vi "CHECK_STOCK.vi"(10 "CURRENT_YEAR_DATA":string, 11 "connection reference":T1) -> ()   [LabVIEW 2015]
uses:
  Controls/CHECK_STOCK.ctl
  <vilib>/addons/database/Connection.llb/Conn ObjectReference.ctl
  <vilib>/Utility/miscctls.llb/LVRowAndColumnUnsignedTypeDef.ctl
  Controls/ITEM_CODE_CLUSTER.ctl
  Controls/STORE_INITAIL_INFORMATION.ctl
  <vilib>/Utility/error.llb/DialogType.ctl
  <vilib>/addons/database/Connection.llb/Conn Execute.vi
  <vilib>/addons/database/Recordset.llb/Rec Destroy - Connection.vi
  <vilib>/addons/database/_DB Variant To Data/Database Variant To Data.xnode
  <vilib>/addons/database/NI_Database_API.lvlib
  <vilib>/addons/database/Connection.llb/DB Tools Open Connec (String).vi
panel:
  out "COUNTER":i32
  out "Find Array":i32[](array[numeric])
  in  "Next Button":bool
  in  "SEARCH":string
  in  "END_MONTH Button":bool
  out "Array":T2[](array[typedef])
  in  "BOTTON_IMPORT":bool
  in  "BUTTON_EXIT":bool
  in  "Tab Control":enum32{"FROM CHECK STOCK", "TRANSFER"}(tab)
  in  "PRODUCT":string(combo)
  in  "INITAIL DATE FROM":string(combo) caption="DATE FROM"
  in  "TO":string(combo)
  in  "TRANFER_DATE_FROM":timestamp caption="DATE (FROM)" format="%<%Y>T"
  in  "(TO)":timestamp format="%<%Y>T"
  out "Table":string[][](table)
  # "CHECK STOCK"
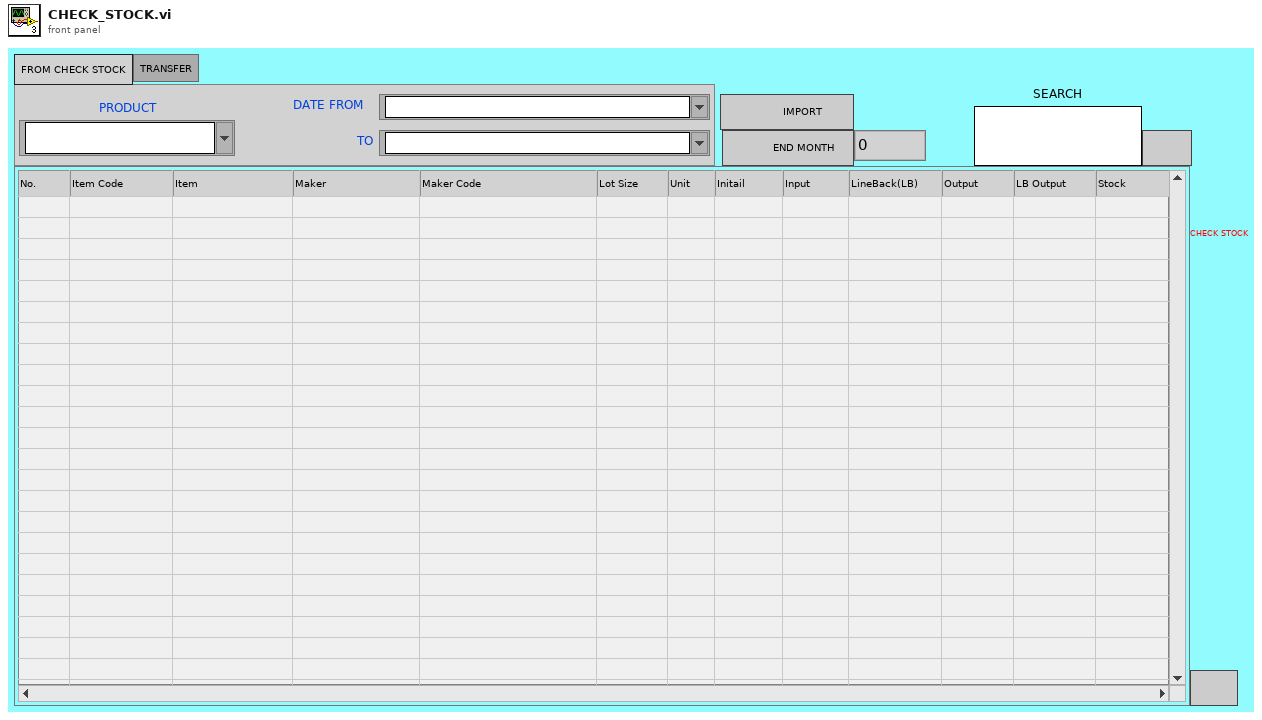
[diagram p1: front panel]
types:
  T1 = typedef "NI_Database_API.lvlib/Conn ObjectReference.ctl" = refnum<k1>
  T2 = typedef "CHECK_STOCK.ctl" = cluster{"ITEM_CODE":string, "PART_NAME":string, "MAKER":string, "PART_NO":string, "LOT_SIZE":dbl, "UNIT":string, "INITAIL":dbl, "INPUT":dbl, "OUTPUT":dbl, "LINEBACK":dbl, "LINEBACK_OUTPUT":dbl, "STOCK":dbl}
  T3 = typedef "LVRowAndColumnUnsignedTypeDef.ctl" = cluster{"Row":u32, "Column":u32}
  T4 = typedef "ITEM_CODE_CLUSTER.ctl" = cluster{"ITEM_CODE":string, "INVOICE_NO":string, "INVOICE_DATE":timestamp, "LOT_MAKER":string, "QUANTITY":dbl, "INVOICE_ECODE":string, "INPUT_NO":string, "INPUT_DATE":timestamp, "INPUT_ECODE":string, "LINEBACK_NO":string, "LINEBACK_DATE":timestamp, "LINEBACK_ECODE":string, "OUTPUT_NO":string, "OUTPUT_DATE":timestamp, "OUTPUT_ECODE":string, "DESTINATION":string}
  T5 = typedef "STORE_INITAIL_INFORMATION.ctl" = cluster{"DATE":timestamp, "PRODUCT":string, "NO":string, "ECODE":string}
  T6 = typedef "NI_Database_API.lvlib/Rec ObjectReference.ctl" = refnum<k1>
  T7 = typedef "DialogType.ctl" = u16
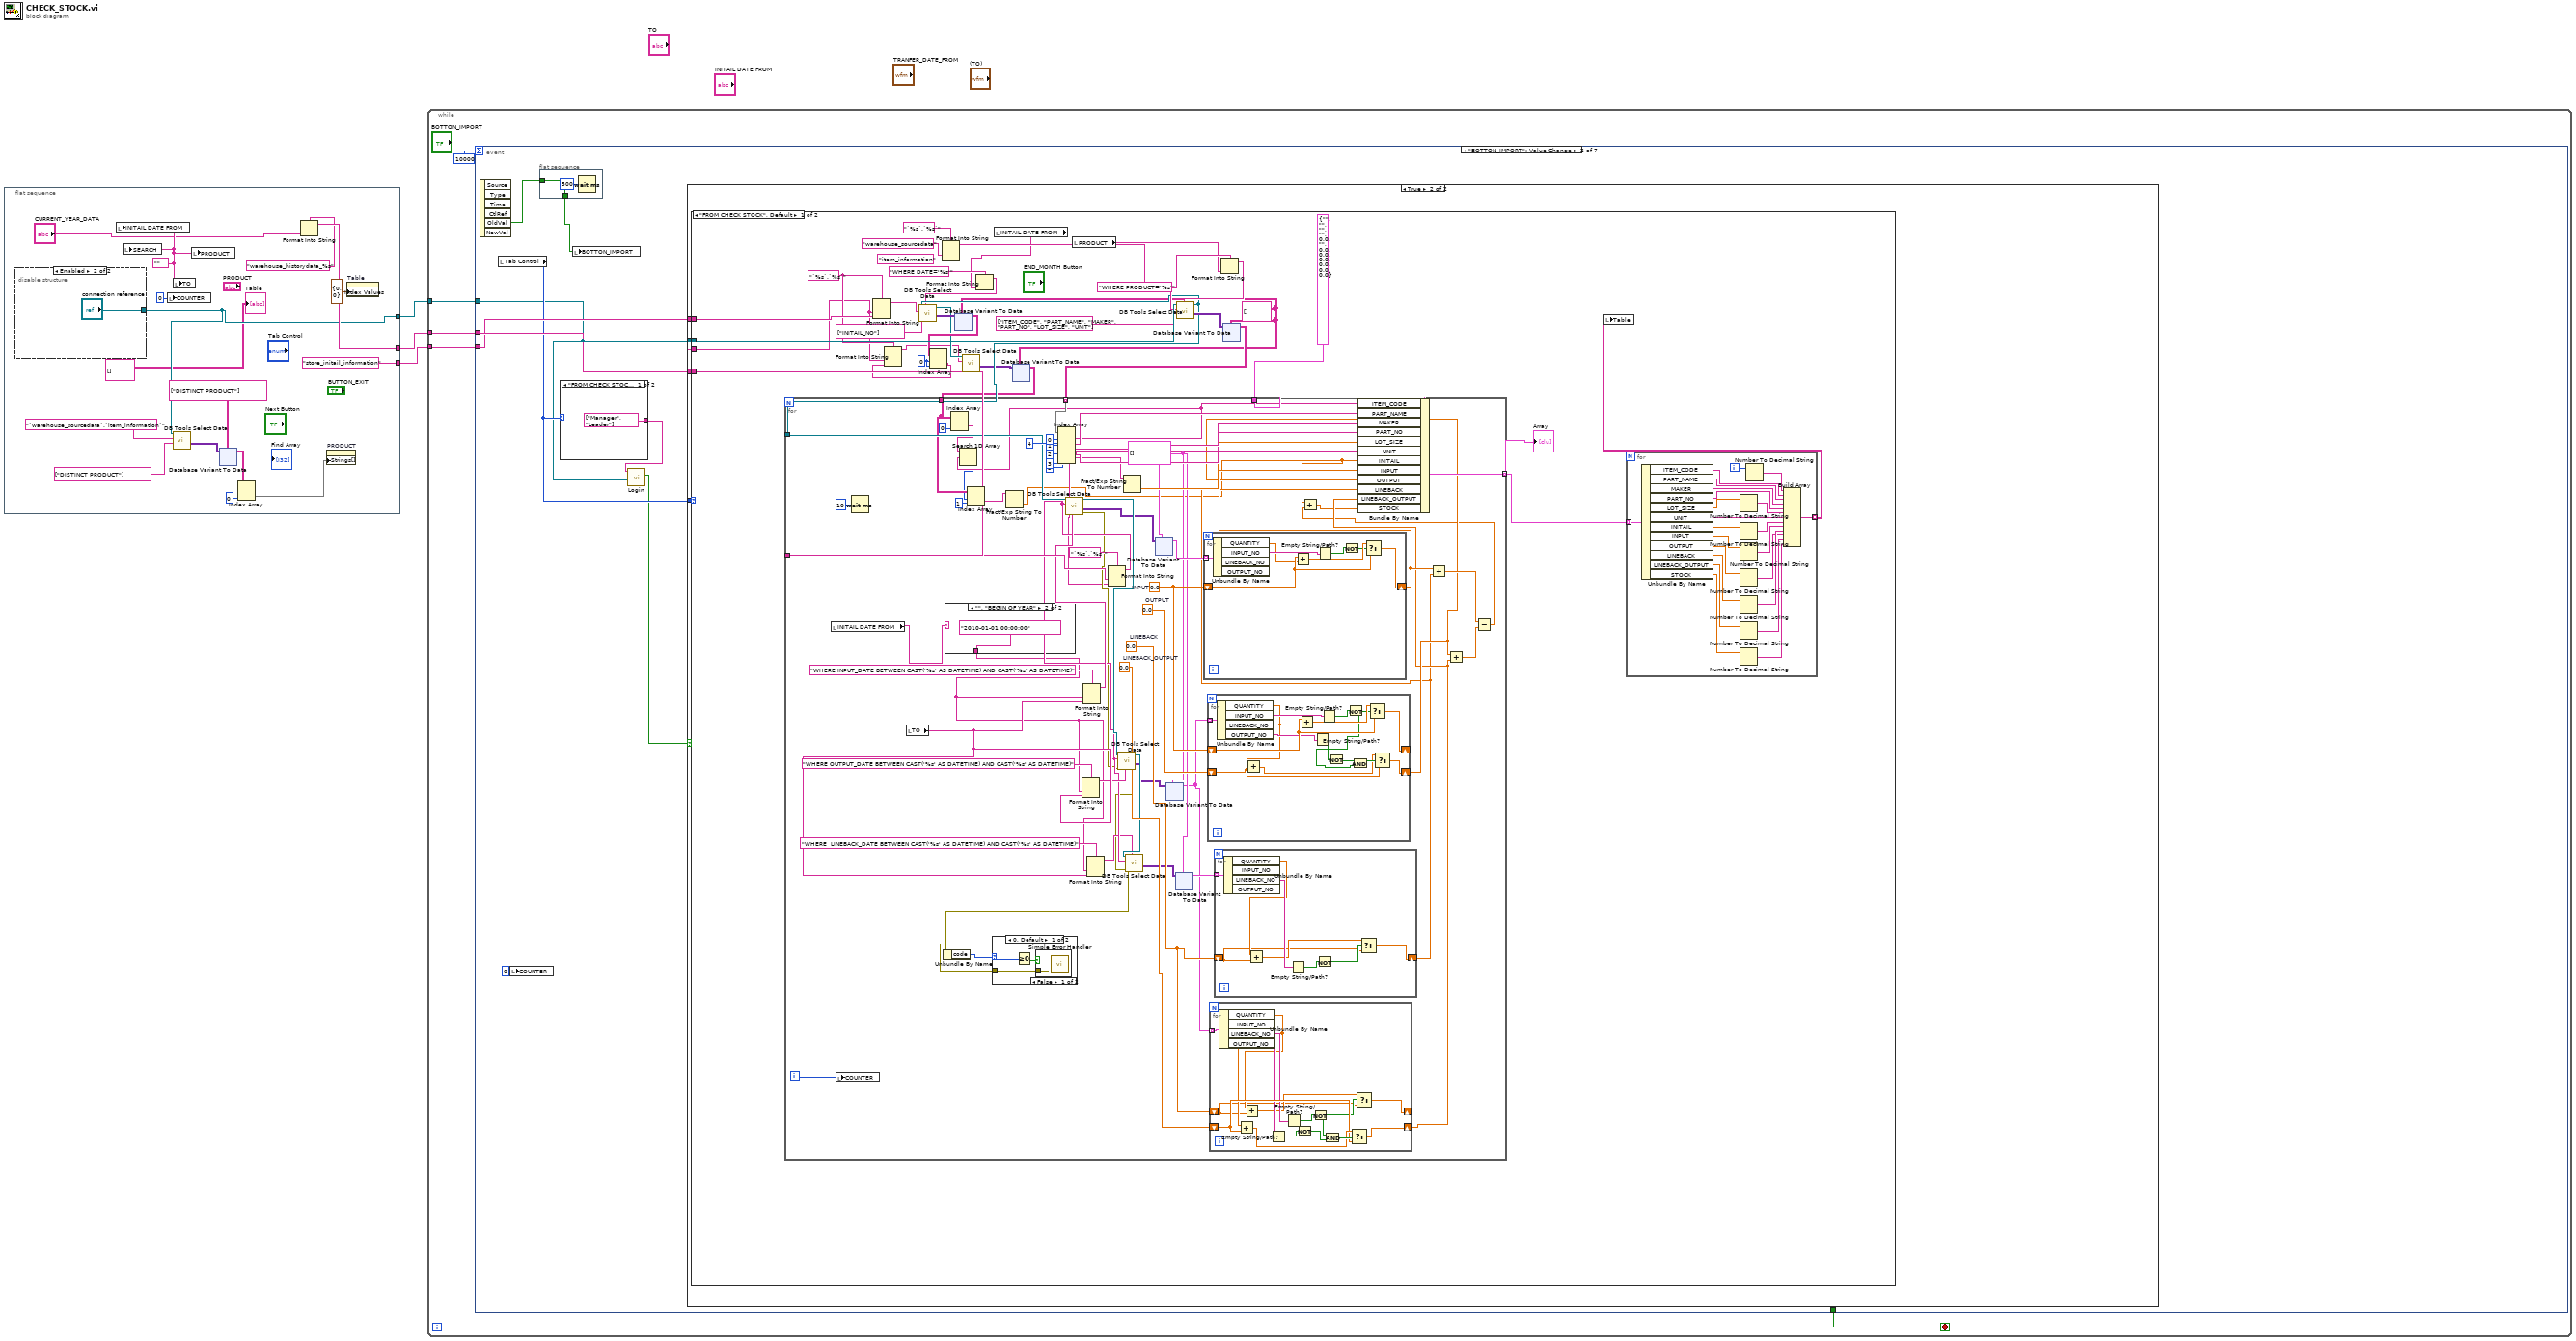
[diagram p0: block diagram]
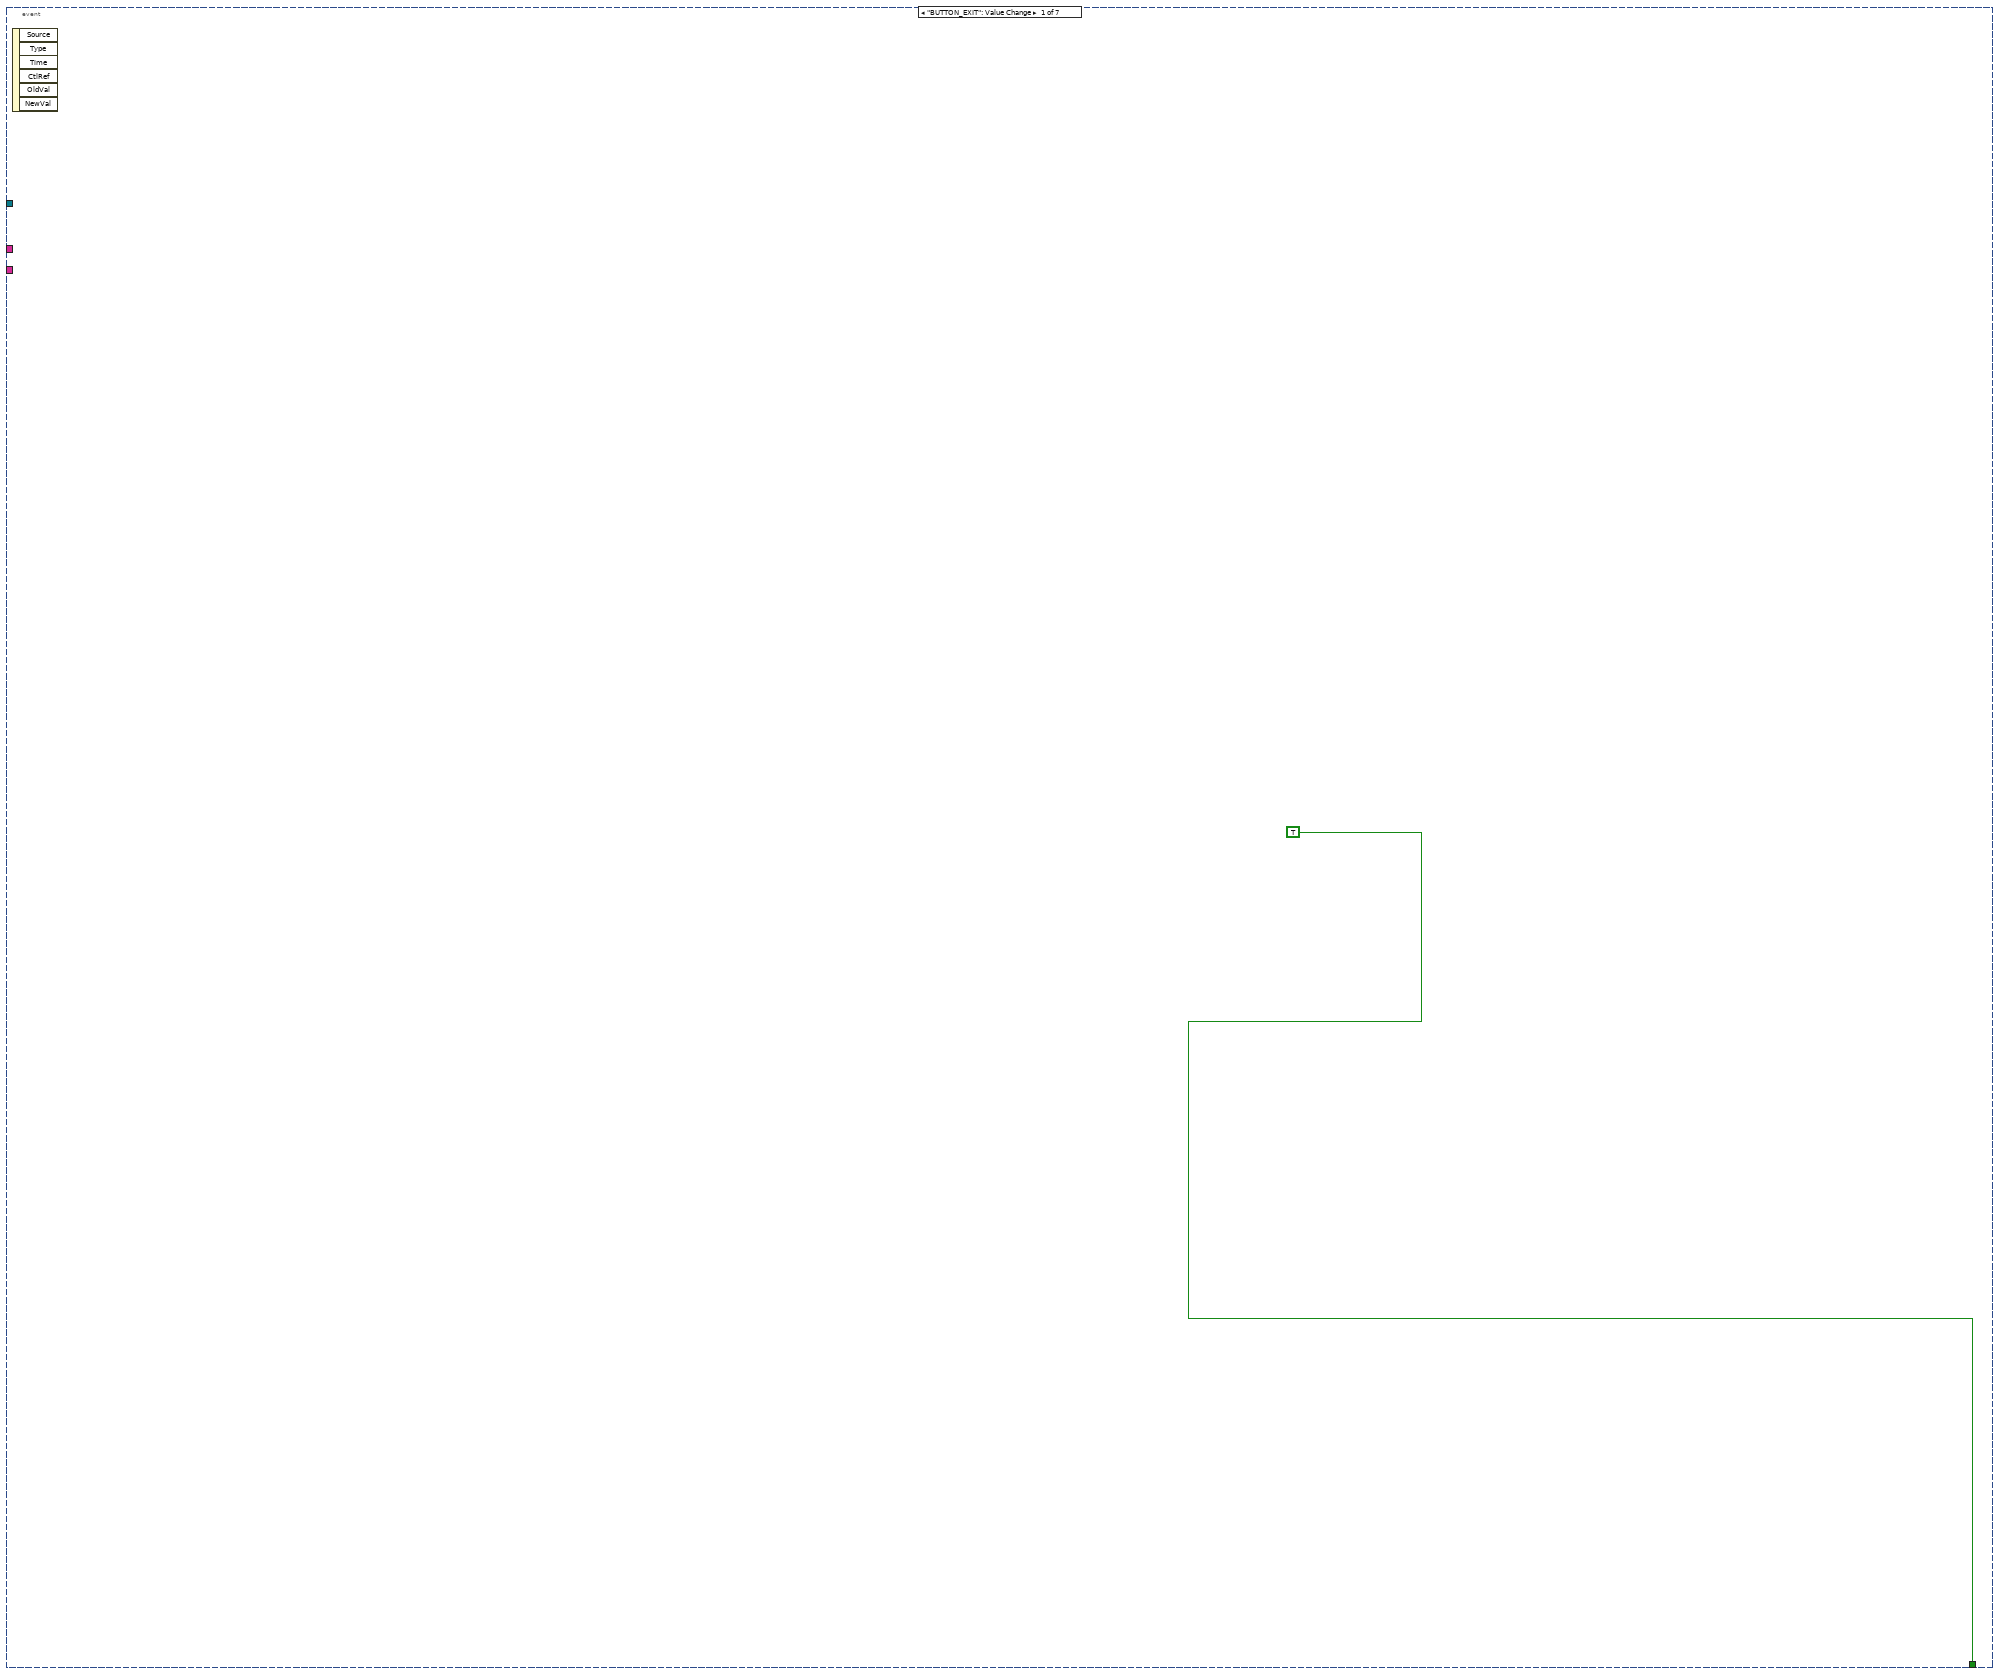
[diagram p2: hidden frame]
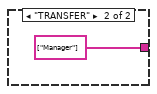
[diagram p3: hidden frame]
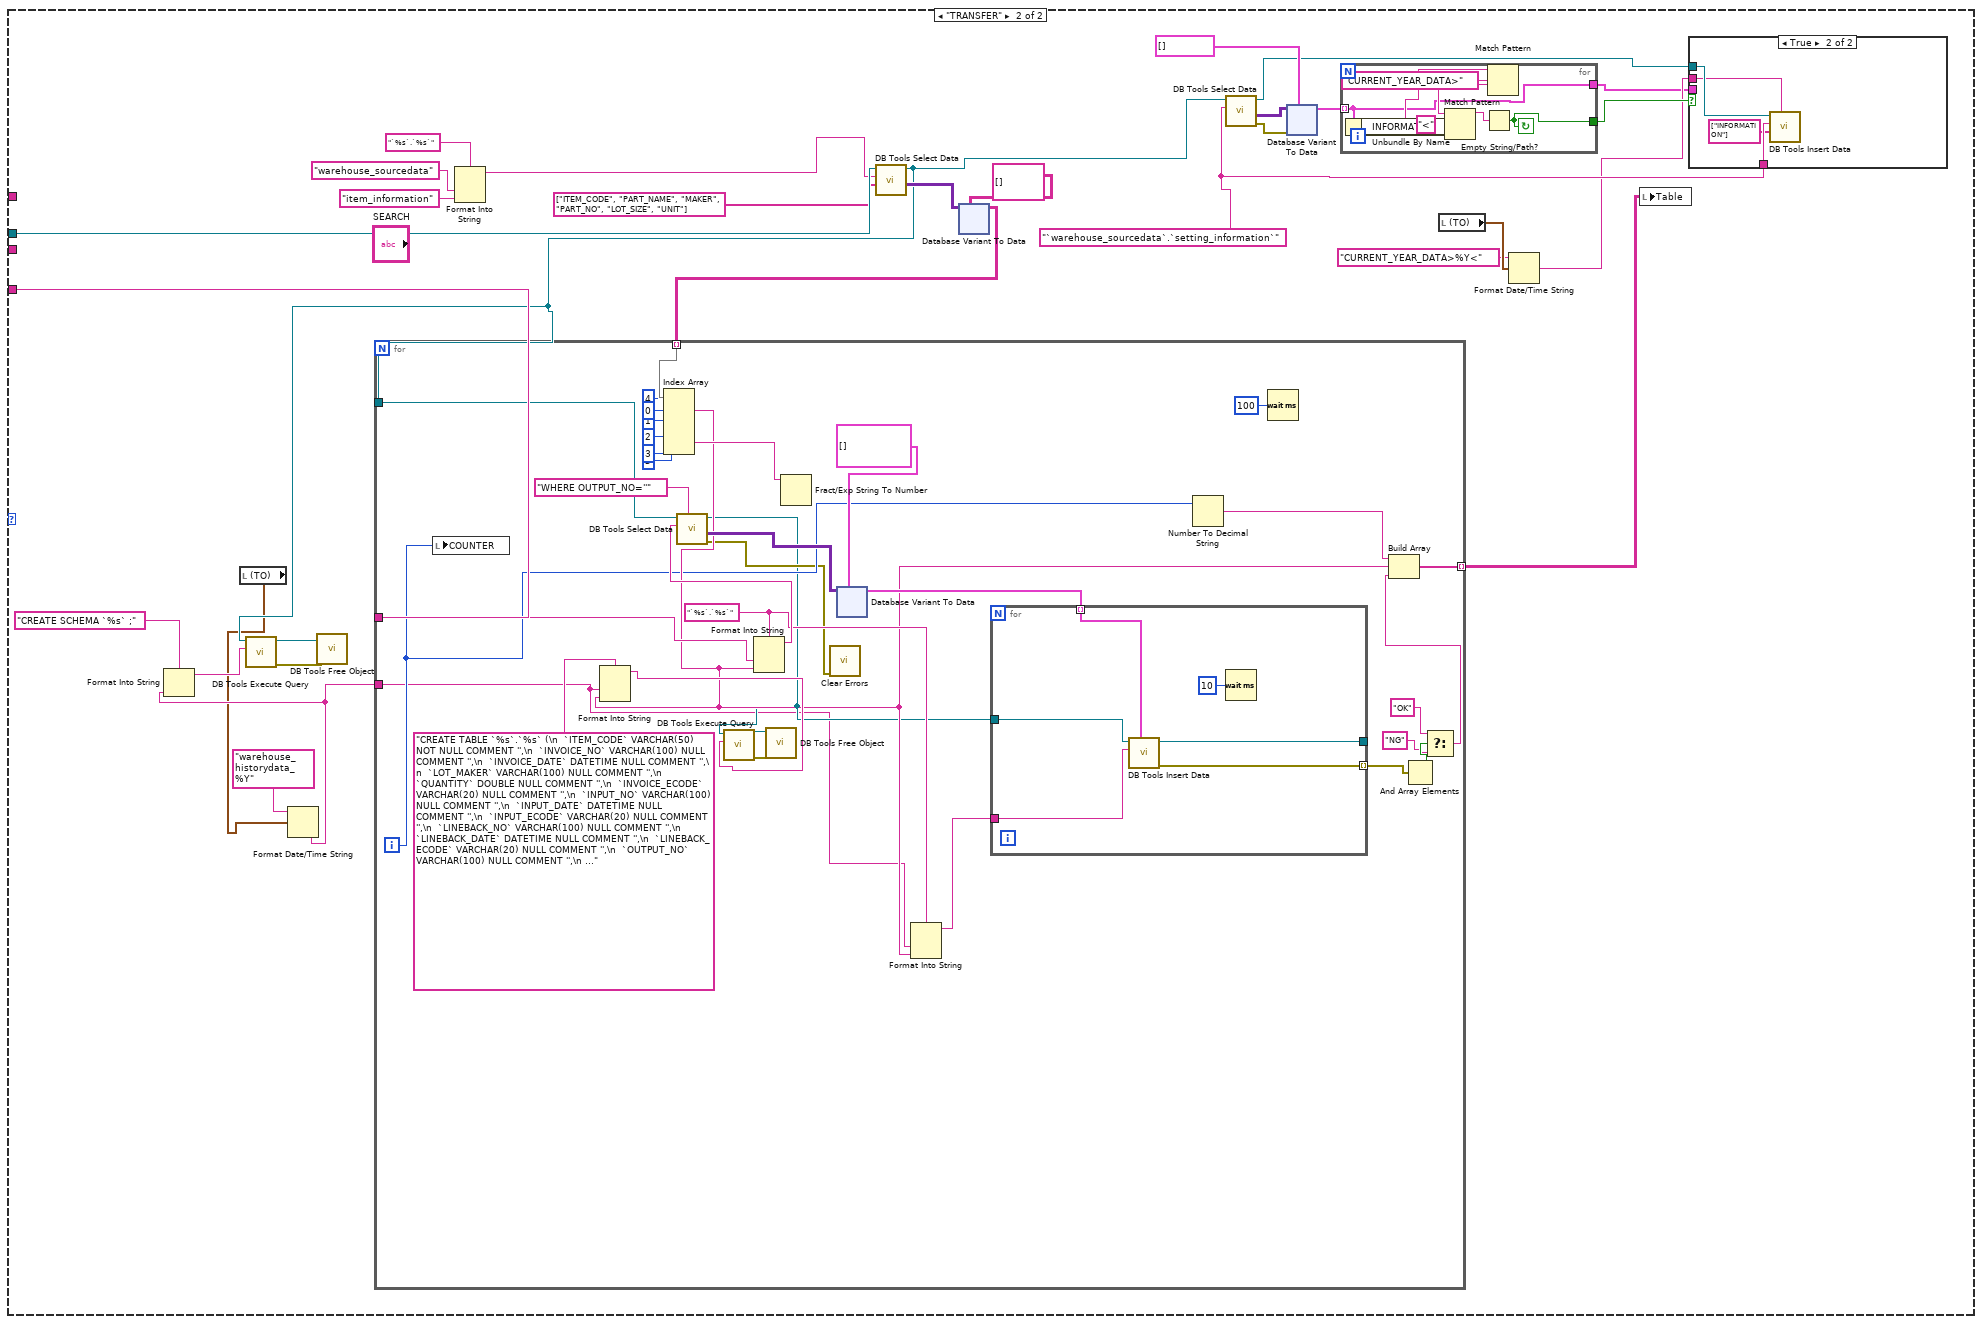
[diagram p8: hidden frame]
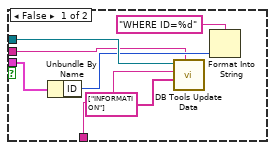
[diagram p9: hidden frame]
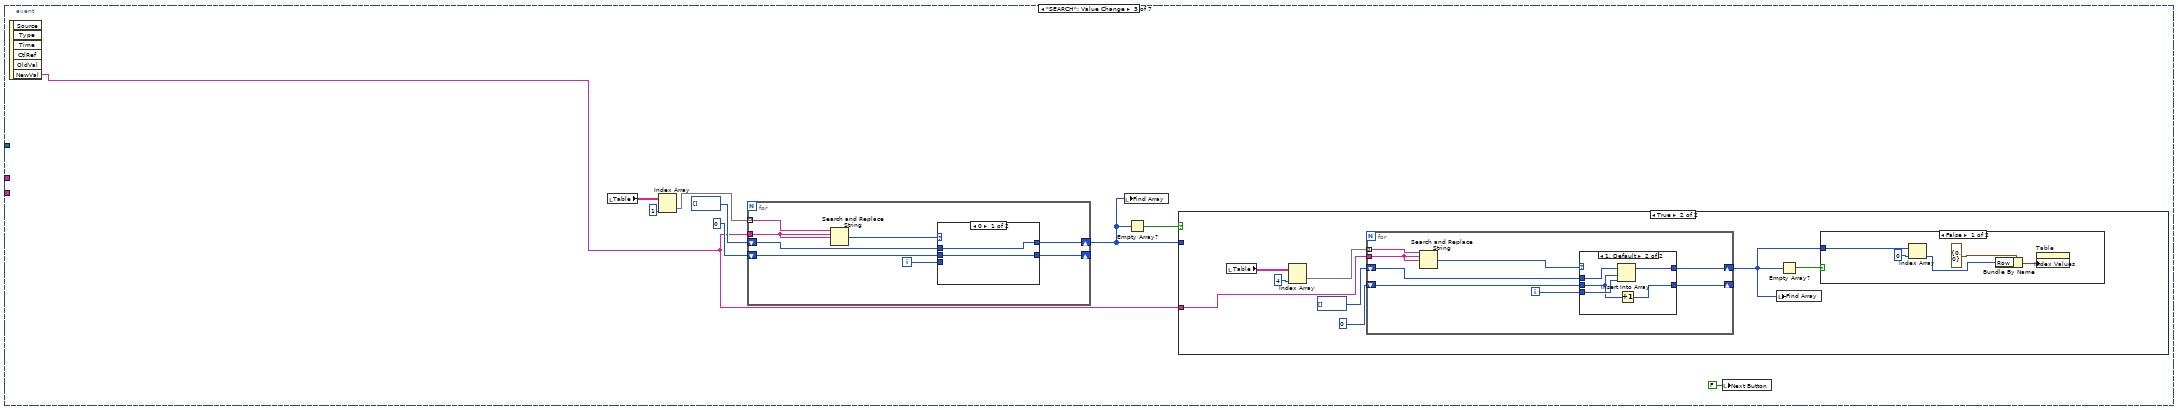
[diagram p10: hidden frame]
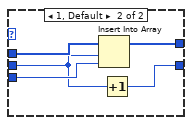
[diagram p11: hidden frame]
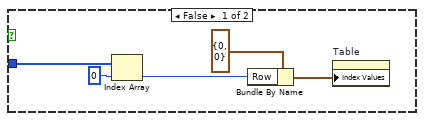
[diagram p12: hidden frame]
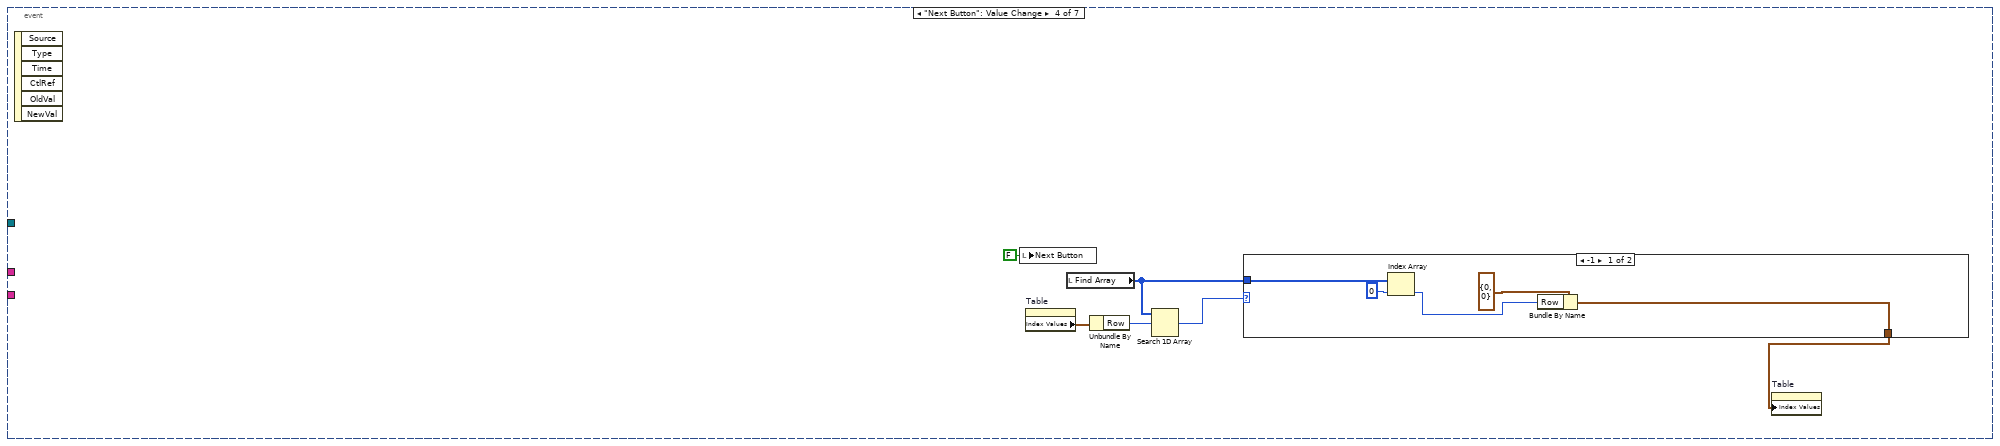
[diagram p15: hidden frame]
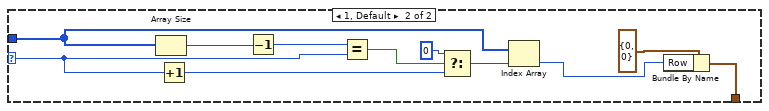
[diagram p16: hidden frame]
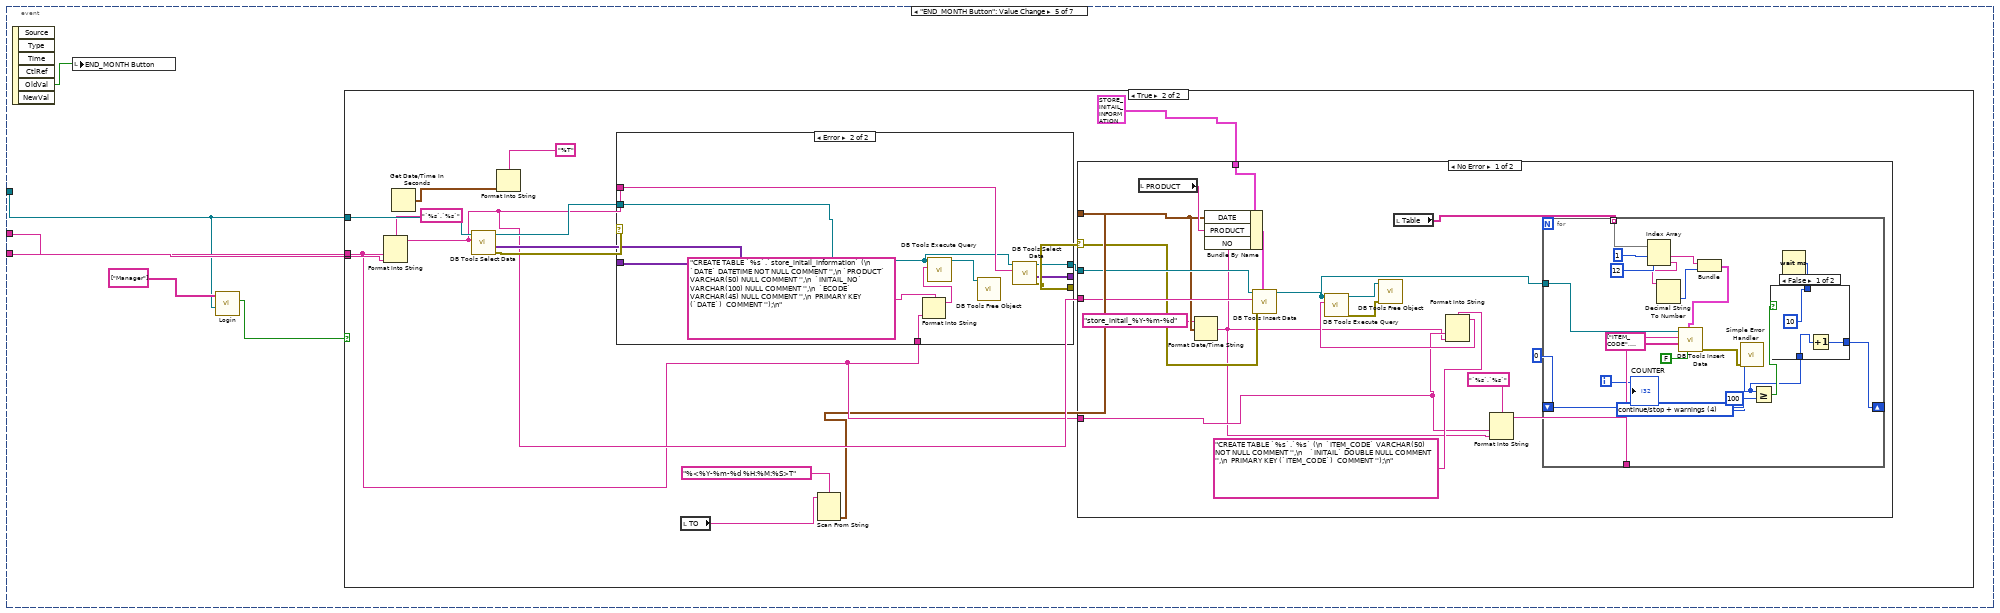
[diagram p17: hidden frame]
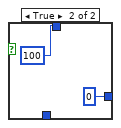
[diagram p19: hidden frame]
diagram:
  n1 = flat-sequence {
    tunnel: [w17] -> w3
    tunnel: [w19] -> w2
    tunnel: ["store_initail_information" ("table")] -> w1
    frame #0 {
      w7 = "" ("TO")
      n2 = disable-structure shown="Enabled" {
        disable-tunnel: [w21 "connection reference"] -> w17
        frame Disabled {
          n3 = call-poly <vilib>:"DB Tools Open Connection.vi"("password"="871994" ("userID"), "userID"="hoangbao2106", "connection information"="database" ("userID")) -> ("connection reference"=w21:T1)  [unwired: 5 in, 1 out]
        }
        frame Enabled {
        }
      }
      n4 = local write "INITAIL DATE FROM"(w7) -> ()
      n5 = local write "SEARCH"(w7) -> ()
      n6 = local write "COUNTER"(0 ("COUNTER")) -> ()
      n7 = call <vilib>:"DB Tools Select Data.vi"("columns"=string[] ["DISTINCT PRODUCT"], "table"="`warehouse_sourcedata`.`item_information`", "connection reference"=w17) -> ("data"=w14:variant[][])  [unwired: 3 in, 2 out]
      n8 = local write "TO"(w7) -> ()
      n9 = local write "PRODUCT"(w7) -> ()
      n10 = xnode "Database Variant To Data"("database variant"=w14, "type"=string[][] [["DISTINCT PRODUCT"]] ("columns")) -> ("data"=w12:string[][])  [unwired: 1 in, 1 out]
      n11 = Index Array(array=w12, index (col)=0 ("disabled index (col)")) -> (element=w10:string[])  [unwired: 1 in]
      n12 = Format Into String(format string="warehouse_historydata_%s" ("table"), "CURRENT_YEAR_DATA") -> (resulting string=w19:string)  [unwired: 2 in, 1 out]
      n13 = property on="PRODUCT" class="CmbBox"("Strings[]"=w10) -> ()  [unwired: 2 in, 2 out]
      n14 = property on="Table" class="Tbl (strict)"("Index Values"=T3 {"Row"=0, "Column"=0}) -> ()  [unwired: 2 in, 2 out]
      "Table" <- string[][] []
    }
  }
  n15 = while {
    tunnel: w3 -> [w72]
    tunnel: w2 -> [w71]
    tunnel: w1 -> [w69]
    stop <- w73 stop-if-true
    n16 = event shown="[1] \"BOTTON_IMPORT\": Value Change" {
      selector: _ -> [_ _ _ _ _ _ _]
      dyn-events: _ -> [_ _ _ _ _ _ _]
      timeout: 10000 -> [_ _ _ _ _ _ _]
      tunnel: [TRUE _ _ _ _ _ _] -> w73
      tunnel: w72 -> [_ w78 _ _ w2910 w3004 _]
      tunnel: w71 -> [_ w83 _ _ w2914 w2997 _]
      tunnel: w69 -> [_ w82 _ _ w2915 w3006 _]
      event "BUTTON_EXIT": Value Change {
        n17 = event-data() -> ()  [unwired: 1 in, 6 out]
      }
      event "BOTTON_IMPORT": Value Change {
        n18 = event-data() -> ("OldVal"=w77:bool)  [unwired: 1 in, 5 out]
        n19 = local read "Tab Control"() -> (w81:enum32{"FROM CHECK STOCK", "TRANSFER"})
        n20 = local write "COUNTER"(0 ("COUNTER")) -> ()
        n21 = flat-sequence {
          tunnel: [w85] -> w76
          tunnel: w77 -> [w85]
          frame #0 {
            n22 = Wait (ms)(milliseconds to wait=u32 500) -> ()  [unwired: 1 out]
          }
        }
        n23 = case shown="\"FROM CHECK STOCK\", Default" w81 {
          tunnel: [string[] ["Manager", "Leader"] ("Permission") string[] ["Manager"] ("Permission")] -> w80
          frame "FROM CHECK STOCK", Default {
          }
          frame "TRANSFER" {
          }
        }
        n24 = local write "BOTTON_IMPORT"(w76) -> ()
        n25 = call "Login.vi"("connection reference"=w78, "Permission"=w80) -> ("OK"=w79:bool)  [unwired: 8 in, 1 out]
        n26 = case shown="True" w79 {
          tunnel: w81 -> [_ w91]
          tunnel: w78 -> [_ w90]
          tunnel: w83 -> [_ w89]
          tunnel: w82 -> [_ w88]
          frame False {
          }
          frame True {
            n27 = case shown="\"FROM CHECK STOCK\", Default" w91 {
              tunnel: w90 -> [w124 w2098]
              tunnel: w89 -> [w116 w2090]
              tunnel: w89 -> [w98 _]
              tunnel: w88 -> [w109 _]
              frame "FROM CHECK STOCK", Default {
                w101 = 0 ("index (row)")
                w99 = "`%s`.`%s`" ("table")
                w94 = string[][] []
                n28 = Format Into String(format string=w99, w98, w109) -> (resulting string=w108:string)  [unwired: 2 in, 1 out]
                n29 = Format Into String(format string="`%s`.`%s`" ("table"), "warehouse_sourcedata" ("table"), "item_information" ("table")) -> (resulting string=w120:string)  [unwired: 2 in, 1 out]
                n30 = local read "INITAIL DATE FROM"() -> (w92:string)
                n31 = Format Into String(format string="WHERE DATE='%s'" ("condition"), w92) -> (resulting string=w104:string)  [unwired: 2 in, 1 out]
                n32 = local read "PRODUCT"() -> (w110:string)
                n33 = Format Into String(format string="WHERE PRODUCT='%s'" ("condition"), w110) -> (resulting string=w111:string)  [unwired: 2 in, 1 out]
                n34 = call <vilib>:"DB Tools Select Data.vi"("condition"=w111, "columns"=string[] ["ITEM_CODE", "PART_NAME", "MAKER", "PART_NO", "LOT_SIZE", "UNIT"], "table"=w120, "connection reference"=w124) -> ("data"=w118:variant[][], "connection reference out"=w107:T1)  [unwired: 2 in, 1 out]
                n35 = call <vilib>:"DB Tools Select Data.vi"("condition"=w104, "columns"=string[] ["INITAIL_NO"], "table"=w108, "connection reference"=w107) -> ("data"=w103:variant[][], "connection reference out"=w100:T1)  [unwired: 2 in, 1 out]
                n36 = xnode "Database Variant To Data"("database variant"=w103, "type"=w94) -> ("data"=w102:string[][])  [unwired: 1 in, 1 out]
                n37 = Index Array(array=w102, index (row)=w101, index (col)=w101) -> (element=w97:string)
                n38 = Format Into String(format string=w99, w98, w97) -> (resulting string=w96:string)  [unwired: 2 in, 1 out]
                n39 = call <vilib>:"DB Tools Select Data.vi"("table"=w96, "connection reference"=w100) -> ("data"=w95:variant[][])  [unwired: 4 in, 2 out]
                n40 = xnode "Database Variant To Data"("database variant"=w95, "type"=w94) -> ("data"=w93:string[][])  [unwired: 1 in, 1 out]
                n41 = xnode "Database Variant To Data"("database variant"=w118, "type"=w94) -> ("data"=w115:string[][])  [unwired: 1 in, 1 out]
                n42 = for {
                  tunnel: w115 -> [w342] mode=indexing
                  tunnel: w107 -> [w334]
                  tunnel: T2 {"ITEM_CODE"="", "PART_NAME"="", "MAKER"="", "PART_NO"="", "LOT_SIZE"=0.0, "UNIT"="", "INITAIL"=0.0, "INPUT"=0.0, "OUTPUT"=0.0, "LINEBACK"=0.0, "LINEBACK_OUTPUT"=0.0, "STOCK"=0.0} ("INVENTORY_Cluster") -> [w335]
                  tunnel: w116 -> [w332]
                  tunnel: [w322] -> w114 mode=indexing
                  tunnel: w93 -> [w292]
                  i -> [w284]
                  w317 = 0.0  # LINEBACK_OUTPUT
                  w318 = 0.0  # LINEBACK
                  w319 = 0.0  # OUTPUT
                  w320 = 0.0  # INPUT
                  w301 = T4[] []
                  n43 = local read "INITAIL DATE FROM"() -> (w286:string)
                  n44 = local write "COUNTER"(w284) -> ()
                  n45 = Wait (ms)(milliseconds to wait=u32 10) -> ()  [unwired: 1 out]
                  n46 = local read "TO"() -> (w308:string)
                  n47 = case shown="\"\", \"BEGIN OF YEAR\"" w286 {
                    selector: w286 -> [w343 _]
                    tunnel: [w343 "2010-01-01 00:00:00"] -> w285
                    frame "False", Default {
                    }
                    frame "", "BEGIN OF YEAR" {
                    }
                  }
                  n48 = Index Array(array=w292, index (col)=0 ("disabled index (col)")) -> (element=w294:string[])  [unwired: 1 in]
                  n49 = Index Array(array=w342, index #1=0 ("index"), index #2=1 ("index"), index #3=2 ("index"), index #4=3 ("index"), index #5=4 ("index"), index #6=5 ("index")) -> (element #1=w293:string, element #2=w331:string, element #3=w330:string, element #4=w329:string, element #5=w327:string, element #6=w328:string)
                  n50 = Search 1D Array(1D array=w294, element=w293) -> (index of element=w291:i32)  [unwired: 1 in]
                  n51 = Index Array(array=w292, index (row)=w291, index (col)=1 ("disabled index (col)")) -> (element=w289:string)
                  n52 = Fract/Exp String To Number(string=w289) -> (number=w282:dbl)  [unwired: 3 in, 1 out]
                  n53 = Format Into String(format string="WHERE OUTPUT_DATE BETWEEN CAST('%s' AS DATETIME) AND CAST('%s' AS DATETIME)" ("table"), w285, w308) -> (resulting string=w307:string)  [unwired: 2 in, 1 out]
                  n54 = Format Into String(format string="WHERE INPUT_DATE BETWEEN CAST('%s' AS DATETIME) AND CAST('%s' AS DATETIME)" ("table"), w285, w308) -> (resulting string=w312:string)  [unwired: 2 in, 1 out]
                  n55 = Format Into String(format string="WHERE  LINEBACK_DATE BETWEEN CAST('%s' AS DATETIME) AND CAST('%s' AS DATETIME)" ("table"), w285, w308) -> (resulting string=w304:string)  [unwired: 2 in, 1 out]
                  n56 = Format Into String(format string="`%s`.`%s`" ("table"), w332, w293) -> (resulting string=w305:string)  [unwired: 2 in, 1 out]
                  n57 = call <vilib>:"DB Tools Select Data.vi"("condition"=w312, "table"=w305, "connection reference"=w334) -> ("error out"=w297:errorcluster, "data"=w303:variant[][], "connection reference out"=w311:T1)  [unwired: 3 in]
                  n58 = call <vilib>:"DB Tools Select Data.vi"("condition"=w307, "error in (no error)"=w297, "table"=w305, "connection reference"=w311) -> ("error out"=w296:errorcluster, "data"=w302:variant[][], "connection reference out"=w306:T1)  [unwired: 2 in]
                  n59 = Fract/Exp String To Number(string=w327) -> (number=w326:dbl)  [unwired: 3 in, 1 out]
                  n60 = call <vilib>:"DB Tools Select Data.vi"("condition"=w304, "error in (no error)"=w296, "table"=w305, "connection reference"=w306) -> ("error out"=w287:errorcluster, "data"=w300:variant[][])  [unwired: 2 in, 1 out]
                  n61 = Unbundle By Name(w287) -> ("code"=w288:i32)
                  n62 = case shown="0, Default" w288 {
                    selector: w288 -> [w347 _]
                    tunnel: w287 -> [w346 _]
                    frame 0, Default {
                      n63 = Greater Or Equal To 0?(x=w347) -> (x >= 0?=w345:bool)
                      n64 = case shown="False" w345 {
                        tunnel: w346 -> [w348 _]
                        frame False {
                          n65 = call <vilib>:"Simple Error Handler.vi"("error in (no error)"=w348) -> ()  [unwired: 4 in, 5 out]
                        }
                        frame True {
                        }
                      }
                    }
                    frame -2147217865 {
                    }
                  }
                  n66 = xnode "Database Variant To Data"("database variant"=w303, "type"=w301) -> ("data"=w321:T4[])  [unwired: 1 in, 1 out]
                  n67 = xnode "Database Variant To Data"("database variant"=w302, "type"=w301) -> ("data"=w298:T4[])  [unwired: 1 in, 1 out]
                  n68 = xnode "Database Variant To Data"("database variant"=w300, "type"=w301) -> ("data"=w299:T4[])  [unwired: 1 in, 1 out]
                  n69 = for {
                    tunnel: w321 -> [w1510] mode=indexing
                    shift-right: [w1505] -> w325
                    shift-left: w320 -> [w1506]
                    n70 = Unbundle By Name(w1510) -> ("QUANTITY"=w1504:dbl, "INPUT_NO"=w1508:string)  [unwired: 2 out]
                    n71 = Add(x=w1506, y=w1504) -> (x+y=w1507:dbl)
                    n72 = Empty String/Path?(string/path=w1508) -> (empty?=w1509:bool)
                    n73 = Not(x=w1509) -> (.not. x?=w1503:bool)
                    n74 = Select(t=w1507, s=w1503, f=w1506) -> (s? t:f=w1505:dbl)
                  }
                  n75 = for {
                    tunnel: w298 -> [w1502] mode=indexing
                    shift-right: [w1488] -> w316
                    shift-left: w319 -> [w1491]
                    shift-right: [w1496] -> _
                    shift-left: w320 -> [w1498]
                    n76 = Unbundle By Name(w1502) -> ("QUANTITY"=w1490:dbl, "INPUT_NO"=w1500:string, "OUTPUT_NO"=w1493:string)  [unwired: 1 out]
                    n77 = Add(x=w1490, y=w1491) -> (x+y=w1492:dbl)
                    n78 = Add(x=w1498, y=w1490) -> (x+y=w1499:dbl)
                    n79 = Empty String/Path?(string/path=w1493) -> (empty?=w1497:bool)
                    n80 = Empty String/Path?(string/path=w1500) -> (empty?=w1501:bool)
                    n81 = Not(x=w1497) -> (.not. x?=w1494:bool)
                    n82 = Not(x=w1501) -> (.not. x?=w1489:bool)
                    n83 = And(x=w1494, y=w1489) -> (x .and. y?=w1495:bool)
                    n84 = Select(t=w1499, s=w1489, f=w1498) -> (s? t:f=w1496:dbl)
                    n85 = Select(t=w1492, s=w1495, f=w1491) -> (s? t:f=w1488:dbl)
                  }
                  n86 = for {
                    shift-right: [w1473] -> w315
                    shift-left: w317 -> [w1474]
                    shift-right: [w1466] -> _
                    shift-left: w318 -> [w1467]
                    tunnel: w298 -> [w1465] mode=indexing
                    n87 = Unbundle By Name(w1465) -> ("QUANTITY"=w1469:dbl, "LINEBACK_NO"=w1472:string, "OUTPUT_NO"=w1471:string)  [unwired: 1 out]
                    n88 = Add(x=w1469, y=w1474) -> (x+y=w1475:dbl)
                    n89 = Add(x=w1469, y=w1467) -> (x+y=w1468:dbl)
                    n90 = Empty String/Path?(string/path=w1471) -> (empty?=w1479:bool)
                    n91 = Empty String/Path?(string/path=w1472) -> (empty?=w1478:bool)
                    n92 = Not(x=w1479) -> (.not. x?=w1477:bool)
                    n93 = Not(x=w1478) -> (.not. x?=w1470:bool)
                    n94 = And(x=w1470, y=w1477) -> (x .and. y?=w1476:bool)
                    n95 = Select(t=w1475, s=w1476, f=w1474) -> (s? t:f=w1473:dbl)
                    n96 = Select(t=w1468, s=w1470, f=w1467) -> (s? t:f=w1466:dbl)
                  }
                  n97 = for {
                    shift-right: [w1481] -> w314
                    shift-left: w318 -> [w1482]
                    tunnel: w299 -> [w1480] mode=indexing
                    n98 = Unbundle By Name(w1480) -> ("QUANTITY"=w1484:dbl, "LINEBACK_NO"=w1486:string)  [unwired: 2 out]
                    n99 = Add(x=w1484, y=w1482) -> (x+y=w1483:dbl)
                    n100 = Empty String/Path?(string/path=w1486) -> (empty?=w1487:bool)
                    n101 = Not(x=w1487) -> (.not. x?=w1485:bool)
                    n102 = Select(t=w1483, s=w1485, f=w1482) -> (s? t:f=w1481:dbl)
                  }
                  n103 = Add(x=w325, y=w314) -> (x+y=w324:dbl)
                  n104 = Add(x=w316, y=w315) -> (x+y=w323:dbl)
                  n105 = Subtract(x=w324, y=w323) -> (x-y=w281:dbl)
                  n106 = Add(x=w282, y=w281) -> (x+y=w280:dbl)
                  n107 = Bundle By Name(cluster=w335, "ITEM_CODE"=w293, "PART_NAME"=w331, "MAKER"=w330, "PART_NO"=w329, "LOT_SIZE"=w326, "UNIT"=w328, "INITAIL"=w282, "INPUT"=w325, "OUTPUT"=w316, "LINEBACK"=w314, "LINEBACK_OUTPUT"=w315, "STOCK"=w280) -> (w322:T2)
                }
                "Array" <- w114
                n108 = for {
                  tunnel: w114 -> [w235] mode=indexing
                  tunnel: [w217] -> w113 mode=indexing
                  i -> [w216]
                  n109 = Unbundle By Name(w235) -> ("ITEM_CODE"=w227:string, "PART_NAME"=w226:string, "MAKER"=w225:string, "PART_NO"=w224:string, "LOT_SIZE"=w228:dbl, "UNIT"=w222:string, "INITAIL"=w229:dbl, "INPUT"=w230:dbl, "OUTPUT"=w231:dbl, "LINEBACK"=w232:dbl, "LINEBACK_OUTPUT"=w233:dbl, "STOCK"=w234:dbl)
                  n110 = Number To Decimal String(number=w228) -> (decimal integer string=w223:string)  [unwired: 1 in]
                  n111 = Number To Decimal String(number=w229) -> (decimal integer string=w221:string)  [unwired: 1 in]
                  n112 = Number To Decimal String(number=w230) -> (decimal integer string=w220:string)  [unwired: 1 in]
                  n113 = Number To Decimal String(number=w231) -> (decimal integer string=w213:string)  [unwired: 1 in]
                  n114 = Number To Decimal String(number=w232) -> (decimal integer string=w214:string)  [unwired: 1 in]
                  n115 = Number To Decimal String(number=w233) -> (decimal integer string=w219:string)  [unwired: 1 in]
                  n116 = Number To Decimal String(number=w234) -> (decimal integer string=w218:string)  [unwired: 1 in]
                  n117 = Number To Decimal String(number=w216) -> (decimal integer string=w215:string)  [unwired: 1 in]
                  n118 = Build Array(w215, w227, w226, w225, w224, w223, w222, w221, w220, w214, w213, w219, w218) -> (w217:string[])
                }
                n119 = local write "Table"(w113) -> ()
              }
              frame "TRANSFER" {
                w2081 = "`warehouse_sourcedata`.`setting_information`" ("table")
                n120 = local read "(TO)"() -> (w2069:timestamp)
                n121 = Format Date/Time String(time format string (%c)="warehouse_historydata_%Y", seconds (now)=w2069) -> (date/time string=w2070:string)  [unwired: 1 in]
                n122 = Format Into String(format string="CREATE SCHEMA `%s` ;" ("SQL query"), w2070) -> (resulting string=w2074:string)  [unwired: 2 in, 1 out]
                n123 = Format Into String(format string="`%s`.`%s`" ("table"), "warehouse_sourcedata" ("table"), "item_information" ("table")) -> (resulting string=w2094:string)  [unwired: 2 in, 1 out]
                n124 = call <vilib>:"DB Tools Select Data.vi"("columns"=string[] ["ITEM_CODE", "PART_NAME", "MAKER", "PART_NO", "LOT_SIZE", "UNIT"], "table"=w2094, "connection reference"=w2098) -> ("data"=w2092:variant[][], "connection reference out"=w2071:T1)  [unwired: 3 in, 1 out]
                n125 = call-poly <vilib>:"DB Tools Execute Query.vi"("SQL query"=w2074, "connection reference"=w2071) -> ("error out"=w2076:errorcluster, "recordset reference"=w2075:T6)  [unwired: 6 in]
                n126 = call-poly <vilib>:"DB Tools Free Object.vi"("error in (no error)"=w2076, "recordset reference"=w2075) -> ()  [unwired: 8 in, 2 out]
                n127 = xnode "Database Variant To Data"("database variant"=w2092, "type"=string[][] []) -> ("data"=w2089:string[][])  [unwired: 1 in, 1 out]
                n128 = for {
                  tunnel: w2089 -> [w2266] mode=indexing
                  tunnel: w2071 -> [w2259]
                  tunnel: w2090 -> [w2258]
                  tunnel: [w2238] -> w2088 mode=indexing
                  tunnel: w2070 -> [w2234]
                  i -> [w2237]
                  w2247 = "`%s`.`%s`" ("table")
                  n129 = local write "COUNTER"(w2237) -> ()
                  n130 = Index Array(array=w2266, index #1=0 ("index"), index #2=1 ("index"), index #3=2 ("index"), index #4=3 ("index"), index #5=4 ("index"), index #6=5 ("index")) -> (element #1=w2240:string, element #5=w2254:string)  [unwired: 4 out]
                  n131 = Format Into String(format string="CREATE TABLE `%s`.`%s` (\n  `ITEM_CODE` VARCHAR(50) NOT NULL COMMENT '',\n  `INVOICE_NO` VARCHAR(100) NULL COMMENT '',\n  `INVOICE_DATE` DATETIME NULL COMMENT '',\n  `LOT_MAKER` VARCHAR(100) NULL COMMENT '',\n  `QUANTITY` DOUBLE NULL COMMENT '',\n  `INVOICE_ECODE` VARCHAR(20) NULL COMMENT '',\n  `INPUT_NO` VARCHAR(100) NULL COMMENT '',\n  `INPUT_DATE` DATETIME NULL COMMENT '',\n  `INPUT_ECODE` VARCHAR(20) NULL COMMENT '',\n  `LINEBACK_NO` VARCHAR(100) NULL COMMENT '',\n  `LINEBACK_DATE` DATETIME NULL COMMENT '',\n  `LINEBACK_ECODE` VARCHAR(20) NULL COMMENT '',\n  `OUTPUT_NO` VARCHAR(100) NULL COMMENT '',\n  `OUTPUT_DATE` DATETIME NULL COMMENT '',\n  `OUTPUT_ECODE` VARCHAR(20) NULL COMMENT '',\n  `DESTINATION` VARCHAR(100) NULL COMMENT '');" ("SQL query"), w2234, w2240) -> (resulting string=w2248:string)  [unwired: 2 in, 1 out]
                  n132 = Format Into String(format string=w2247, w2258, w2240) -> (resulting string=w2257:string)  [unwired: 2 in, 1 out]
                  n133 = call <vilib>:"DB Tools Select Data.vi"("condition"="WHERE OUTPUT_NO=''", "table"=w2257, "connection reference"=w2259) -> ("error out"=w2236:errorcluster, "data"=w2256:variant[][], "connection reference out"=w2235:T1)  [unwired: 3 in]
                  n134 = call-poly <vilib>:"DB Tools Execute Query.vi"("SQL query"=w2248, "connection reference"=w2235) -> ("error out"=w2251:errorcluster, "recordset reference"=w2250:T6)  [unwired: 6 in]
                  n135 = call-poly <vilib>:"DB Tools Free Object.vi"("error in (no error)"=w2251, "recordset reference"=w2250) -> ()  [unwired: 8 in, 2 out]
                  n136 = Fract/Exp String To Number(string=w2254) -> ()  [unwired: 3 in, 2 out]
                  n137 = call <vilib>:"Clear Errors.vi"("error in (no error)"=w2236) -> ()  [unwired: 5 in, 2 out]
                  n138 = xnode "Database Variant To Data"("database variant"=w2256, "type"=T4[] []) -> ("data"=w2252:T4[])  [unwired: 1 in, 1 out]
                  n139 = Format Into String(format string=w2247, w2234, w2240) -> (resulting string=w2246:string)  [unwired: 2 in, 1 out]
                  n140 = for {
                    tunnel: w2252 -> [w2270] mode=indexing
                    tunnel: w2235 -> [w2272]
                    tunnel: w2246 -> [w2271]
                    tunnel: [w2269] -> _
                    tunnel: [w2268] -> w2245 mode=indexing
                    n141 = call <vilib>:"DB Tools Insert Data.vi"("data"=w2270, "table"=w2271, "connection reference"=w2272) -> ("error out"=w2268:errorcluster, "connection reference out"=w2269:T1)  [unwired: 7 in]
                    n142 = Wait (ms)(milliseconds to wait=u32 10) -> ()  [unwired: 1 out]
                  }
                  n143 = Number To Decimal String(number=w2237) -> (decimal integer string=w2241:string)  [unwired: 1 in]
                  n144 = Wait (ms)(milliseconds to wait=u32 100) -> ()  [unwired: 1 out]
                  n145 = And Array Elements(Boolean array=w2245) -> (logical AND=w2244:bool)
                  n146 = Select(t="OK", s=w2244, f="NG") -> (s? t:f=w2239:string)
                  n147 = Build Array(w2241, w2240, w2239) -> (w2238:string[])
                }
                n148 = call <vilib>:"DB Tools Select Data.vi"("table"=w2081, "connection reference"=w2071) -> ("error out"=w2086:errorcluster, "data"=w2087:variant[][], "connection reference out"=w2082:T1)  [unwired: 4 in]
                n149 = xnode "Database Variant To Data"("database variant"=w2087, "error in (no error)"=w2086, "type"=cluster{"ID":i32, "INFORMATION":string}[] []) -> ("data"=w2084:cluster{"ID":i32, "INFORMATION":string}[])  [unwired: 1 out]
                n150 = for {
                  tunnel: w2084 -> [w2110] mode=indexing
                  tunnel: [w2111] -> w2083
                  tunnel: [w2110] -> w2077
                  stop <- w2111 continue-if-true
                  n151 = Unbundle By Name(w2110) -> ("INFORMATION"=w2112:string)
                  n152 = Match Pattern(string=w2112, regular expression="CURRENT_YEAR_DATA>") -> (after substring=w2115:string)  [unwired: 1 in, 3 out]
                  n153 = Match Pattern(string=w2115, regular expression="<") -> (before substring=w2113:string)  [unwired: 1 in, 3 out]
                  n154 = Empty String/Path?(string/path=w2113) -> (empty?=w2111:bool)
                }
                n155 = local read "(TO)"() -> (w2080:timestamp)
                n156 = Format Date/Time String(time format string (%c)="CURRENT_YEAR_DATA>%Y<", seconds (now)=w2080) -> (date/time string=w2078:string)  [unwired: 1 in]
                n157 = local write "Table"(w2088) -> ()
                n158 = case shown="True" w2083 {
                  tunnel: w2082 -> [w2105 w2109]
                  tunnel: w2081 -> [w2099 w2108]
                  tunnel: w2078 -> [w2100 w2107]
                  tunnel: w2077 -> [w2104 _]
                  frame False {
                    n159 = Unbundle By Name(w2104) -> ("ID"=w2101:i32)
                    n160 = call <vilib>:"DB Tools Update Data.vi"("data"=w2100, "columns"=string[] ["INFORMATION"], "table"=w2099, "connection reference"=w2105) -> ()  [unwired: 6 in, 2 out]
                    n161 = Format Into String(format string="WHERE ID=%d", w2101) -> ()  [unwired: 2 in, 2 out]
                  }
                  frame True {
                    n162 = call <vilib>:"DB Tools Insert Data.vi"("data"=w2107, "columns"=string[] ["INFORMATION"], "table"=w2108, "connection reference"=w2109) -> ()  [unwired: 6 in, 2 out]
                  }
                }
              }
            }
          }
        }
      }
      event "SEARCH": Value Change {
        n163 = event-data() -> ("NewVal"=w2832:string)  [unwired: 1 in, 5 out]
        n164 = local read "Table"() -> (w2833:string[][])
        n165 = Index Array(array=w2833, index (col)=1 ("disabled index (col)")) -> (element=w2835:string[])  [unwired: 1 in]
        n166 = for {
          tunnel: w2835 -> [w2847] mode=indexing
          tunnel: w2832 -> [w2846]
          shift-right: [w2844] -> w2838
          shift-left: i32[] [] ("Find Array") -> [w2843]
          shift-right: [w2840] -> _
          shift-left: 0 -> [w2841]
          i -> [w2842]
          n167 = Search and Replace String(input string=w2847, search string=w2846, replace string=w2846) -> (number of replacements=w2845:i32)  [unwired: 5 in, 3 out]
          n168 = case shown="0" w2845 {
            tunnel: [w2849 w2852] -> w2844
            tunnel: w2843 -> [w2849 w2854]
            tunnel: w2842 -> [_ w2853]
            tunnel: w2841 -> [w2848 w2851]
            tunnel: [w2848 w2850] -> w2840
            frame 0 {
            }
            frame 1, Default {
              n169 = Insert Into Array(array=w2854, index=w2851, new element=w2853) -> (w2852:i32[])
              n170 = Increment(x=w2851) -> (x+1=w2850:i32)
            }
          }
        }
        n171 = local write "Find Array"(w2838) -> ()
        n172 = Empty Array?(array=w2838) -> (empty?=w2839:bool)
        n173 = case shown="True" w2839 {
          tunnel: w2832 -> [_ w2860]
          tunnel: w2838 -> [w2858 _]
          frame False {
            n174 = Index Array(array=w2858, index=0) -> (element=w2856:i32)
            n175 = Bundle By Name(cluster=T3 {"Row"=0, "Column"=0} ("Index Values"), "Row"=w2856) -> (w2855:T3)
            n176 = property on="Table" class="Tbl (strict)"("Index Values"=w2855) -> ()  [unwired: 2 in, 2 out]
          }
          frame True {
            n177 = local read "Table"() -> (w2866:string[][])
            n178 = Index Array(array=w2866, index (col)=4 ("disabled index (col)")) -> (element=w2863:string[])  [unwired: 1 in]
            n179 = for {
              tunnel: w2863 -> [w2875] mode=indexing
              tunnel: w2860 -> [w2874]
              shift-right: [w2872] -> w2861
              shift-left: i32[] [] ("Find Array") -> [w2871]
              shift-right: [w2868] -> _
              shift-left: 0 -> [w2869]
              i -> [w2870]
              n180 = Search and Replace String(input string=w2875, search string=w2874, replace string=w2874) -> (number of replacements=w2873:i32)  [unwired: 5 in, 3 out]
              n181 = case shown="1, Default" w2873 {
                tunnel: [w2877 w2880] -> w2872
                tunnel: w2871 -> [w2877 w2882]
                tunnel: w2870 -> [_ w2881]
                tunnel: w2869 -> [w2876 w2879]
                tunnel: [w2876 w2878] -> w2868
                frame 0 {
                }
                frame 1, Default {
                  n182 = Insert Into Array(array=w2882, index=w2879, new element=w2881) -> (w2880:i32[])
                  n183 = Increment(x=w2879) -> (x+1=w2878:i32)
                }
              }
            }
            n184 = local write "Find Array"(w2861) -> ()
            n185 = Empty Array?(array=w2861) -> (empty?=w2862:bool)
            n186 = case shown="False" w2862 {
              tunnel: w2861 -> [w2885 _]
              frame False {
                n187 = Index Array(array=w2885, index=0) -> (element=w2884:i32)
                n188 = Bundle By Name(cluster=T3 {"Row"=0, "Column"=0} ("Index Values"), "Row"=w2884) -> (w2883:T3)
                n189 = property on="Table" class="Tbl (strict)"("Index Values"=w2883) -> ()  [unwired: 2 in, 2 out]
              }
              frame True {
              }
            }
          }
        }
        n190 = local write "Next Button"(FALSE ("Next Button")) -> ()
      }
      event "Next Button": Value Change {
        n191 = event-data() -> ()  [unwired: 1 in, 6 out]
        n192 = local write "Next Button"(FALSE ("Next Button")) -> ()
        n193 = property on="Table" class="Tbl (strict)"() -> ("Index Values"=w2889:T3)  [unwired: 2 in, 2 out]
        n194 = local read "Find Array"() -> (w2892:i32[])
        n195 = Unbundle By Name(w2889) -> ("Row"=w2890:u32)
        n196 = Search 1D Array(1D array=w2892, element=w2890) -> (index of element=w2891:i32)  [unwired: 1 in]
        n197 = case shown="-1" w2891 {
          selector: w2891 -> [_ w2906]
          tunnel: w2892 -> [w2897 w2905]
          tunnel: [w2894 w2899] -> w2888
          frame -1 {
            n198 = Index Array(array=w2897, index=u32 0 ("Row")) -> (element=w2895:i32)
            n199 = Bundle By Name(cluster=T3 {"Row"=0, "Column"=0} ("Index Values"), "Row"=w2895) -> (w2894:T3)
          }
          frame 1, Default {
            n200 = Array Size(array=w2905) -> (size(s)=w2908:i32)
            n201 = Increment(x=w2906) -> (x+1=w2900:i32)
            n202 = Decrement(x=w2908) -> (x-1=w2909:i32)
            n203 = Equal?(x=w2909, y=w2906) -> (x = y?=w2907:bool)
            n204 = Select(t=0 ("f"), s=w2907, f=w2900) -> (s? t:f=w2904:i32)
            n205 = Index Array(array=w2905, index=w2904) -> (element=w2902:i32)
            n206 = Bundle By Name(cluster=T3 {"Row"=0, "Column"=0} ("Index Values"), "Row"=w2902) -> (w2899:T3)
          }
        }
        n207 = property on="Table" class="Tbl (strict)"("Index Values"=w2888) -> ()  [unwired: 2 in, 2 out]
      }
      event "END_MONTH Button": Value Change {
        n208 = event-data() -> ("OldVal"=w2913:bool)  [unwired: 1 in, 5 out]
        n209 = local write "END_MONTH Button"(w2913) -> ()
        n210 = call "Login.vi"("connection reference"=w2910, "Permission"=string[] ["Manager"]) -> ("OK"=w2911:bool)  [unwired: 8 in, 1 out]
        n211 = case shown="True" w2911 {
          tunnel: w2910 -> [_ w2929]
          tunnel: w2915 -> [_ w2927]
          tunnel: w2914 -> [_ w2919]
          frame False {
          }
          frame True {
            n212 = Format Into String(format string="`%s`.`%s`", w2919, w2927) -> (resulting string=w2921:string)  [unwired: 2 in, 1 out]
            n213 = Get Date/Time In Seconds() -> (seconds since 1Jan1904=w2930:timestamp)
            n214 = call <vilib>:"DB Tools Select Data.vi"("table"=w2921, "connection reference"=w2929) -> ("error out"=w2926:errorcluster, "data"=w2925:variant[][], "connection reference out"=w2924:T1)  [unwired: 4 in]
            n215 = Format Into String(format string="%T", w2930) -> ()  [unwired: 2 in, 2 out]
            n216 = case shown="Error" w2926 {
              selector: w2926 -> [w2975 _]
              tunnel: w2925 -> [w2977 _]
              tunnel: w2924 -> [w2976 w2982]
              tunnel: w2921 -> [_ w2986]
              tunnel: [w2977 w2985] -> _
              tunnel: [w2976 w2984] -> w2922
              tunnel: [w2975 w2983] -> w2923
              tunnel: w2919 -> [_ w2980]
              frame No Error {
              }
              frame Error {
                n217 = Format Into String(format string="CREATE TABLE `%s`.`store_initail_information` (\n  `DATE` DATETIME NOT NULL COMMENT '',\n `PRODUCT` VARCHAR(50) NULL COMMENT '',\n  `INITAIL_NO` VARCHAR(100) NULL COMMENT '',\n  `ECODE` VARCHAR(45) NULL COMMENT '',\n  PRIMARY KEY (`DATE`)  COMMENT '');\n" ("SQL query"), w2980) -> (resulting string=w2979:string)  [unwired: 2 in, 1 out]
                n218 = call-poly <vilib>:"DB Tools Execute Query.vi"("SQL query"=w2979, "connection reference"=w2982) -> ("recordset reference"=w2978:T6)  [unwired: 6 in, 1 out]
                n219 = call-poly <vilib>:"DB Tools Free Object.vi"("recordset reference"=w2978) -> ()  [unwired: 9 in, 2 out]
                n220 = call <vilib>:"DB Tools Select Data.vi"("table"=w2986, "connection reference"=w2982) -> ("error out"=w2983:errorcluster, "data"=w2985:variant[][], "connection reference out"=w2984:T1)  [unwired: 4 in]
              }
            }
            n221 = local read "TO"() -> (w2917:string)
            n222 = Scan From String(format string="%<%Y-%m-%d %H:%M:%S>T", input string=w2917) -> (output 1=w2916:timestamp)  [unwired: 3 in, 3 out]
            n223 = case shown="No Error" w2923 {
              selector: w2923 -> [w2946 _]
              tunnel: w2922 -> [w2950 _]
              tunnel: w2921 -> [w2949 _]
              tunnel: T5 {"DATE"=timestamp(0 s since 1904-01-01), "PRODUCT"="", "NO"="", "ECODE"=""} -> [w2948 _]
              tunnel: w2916 -> [w2936 _]
              tunnel: w2919 -> [w2940 _]
              frame No Error {
                n224 = local read "PRODUCT"() -> (w2937:string)
                n225 = Format Date/Time String(time format string (%c)="store_initail_%Y-%m-%d", seconds (now)=w2936) -> (date/time string=w2934:string)  [unwired: 1 in]
                n226 = Bundle By Name(cluster=w2948, "DATE"=w2936, "PRODUCT"=w2937, "NO"=w2934) -> (w2947:T5)
                n227 = call <vilib>:"DB Tools Insert Data.vi"("data"=w2947, "error in (no error)"=w2946, "table"=w2949, "connection reference"=w2950) -> ("connection reference out"=w2933:T1)  [unwired: 6 in, 1 out]
                n228 = local read "Table"() -> (w2938:string[][])
                n229 = Format Into String(format string="CREATE TABLE `%s`.`%s` (\n  `ITEM_CODE` VARCHAR(50) NOT NULL COMMENT '',\n    `INITAIL` DOUBLE NULL COMMENT '',\n  PRIMARY KEY (`ITEM_CODE`)  COMMENT '');\n" ("SQL query"), w2940, w2934) -> (resulting string=w2944:string)  [unwired: 2 in, 1 out]
                n230 = call-poly <vilib>:"DB Tools Execute Query.vi"("SQL query"=w2944, "connection reference"=w2933) -> ("error out"=w2942:errorcluster, "recordset reference"=w2943:T6)  [unwired: 6 in]
                n231 = call-poly <vilib>:"DB Tools Free Object.vi"("error in (no error)"=w2942, "recordset reference"=w2943) -> ()  [unwired: 8 in, 2 out]
                n232 = Format Into String(format string="`%s`.`%s`", w2940, w2934) -> (resulting string=w2939:string)  [unwired: 2 in, 1 out]
                n233 = for {
                  tunnel: w2933 -> [w2969]
                  tunnel: w2939 -> [w2968]
                  tunnel: w2938 -> [w2967] mode=indexing
                  shift-right: [w2960] -> _
                  shift-left: 0 -> [w2959]
                  i -> [w2963]
                  w2958 = T7 4 items=["no dialog", "OK message", "continue or stop message", "OK message + warnings", "continue/stop + warnings"] ("type of dialog (OK msg:1)")
                  n234 = Index Array(array=w2967, index #1=1 ("index"), index #2=12 ("index")) -> (element #1=w2956:string, element #2=w2952:string)
                  n235 = Decimal String To Number(string=w2952) -> (number=w2955:i32)  [unwired: 2 in, 1 out]
                  n236 = Bundle(w2956, w2955) -> (w2951:cluster{string, i32})  [unwired: 1 in]
                  n237 = call <vilib>:"DB Tools Insert Data.vi"("flatten cluster? (F)"=FALSE, "data"=w2951, "columns"=string[] ["ITEM_CODE", "INITAIL"], "table"=w2968, "connection reference"=w2969) -> ("error out"=w2965:errorcluster)  [unwired: 5 in, 1 out]
                  n238 = call <vilib>:"Simple Error Handler.vi"("type of dialog (OK msg:1)"=w2958, "error in (no error)"=w2965) -> ()  [unwired: 3 in, 5 out]
                  n239 = Greater Or Equal?(x=w2959, y=100) -> (x >= y?=w2961:bool)
                  n240 = case shown="False" w2961 {
                    tunnel: [u32 10 ("milliseconds to wait") u32 100 ("milliseconds to wait")] -> w2964
                    tunnel: [w2971 0] -> w2960
                    tunnel: w2959 -> [w2970 _]
                    frame False {
                      n241 = Increment(x=w2970) -> (x+1=w2971:i32)
                    }
                    frame True {
                    }
                  }
                  n242 = Wait (ms)(milliseconds to wait=w2964) -> ()  [unwired: 1 out]
                  "COUNTER" <- w2963
                }
              }
              frame Error {
              }
            }
          }
        }
      }
      event "PRODUCT": Value Change {
        w2995 = "%Y-%m-%d %H:%M:%S" ("time format string (%c)")
        n243 = event-data() -> ()  [unwired: 1 in, 6 out]
        n244 = local read "PRODUCT"() -> (w3002:string)
        n245 = Format Into String(format string="`%s`.`%s`", w2997, w3006) -> (resulting string=w3005:string)  [unwired: 2 in, 1 out]
        n246 = Format Into String(format string="WHERE PRODUCT='%s' ORDER BY `DATE` ASC", w3002) -> (resulting string=w3001:string)  [unwired: 2 in, 1 out]
        n247 = call <vilib>:"DB Tools Select Data.vi"("condition"=w3001, "table"=w3005, "connection reference"=w3004) -> ("data"=w3000:variant[][])  [unwired: 3 in, 2 out]
        n248 = xnode "Database Variant To Data"("database variant"=w3000, "type"=T5[] []) -> ("data"=w2998:T5[])  [unwired: 1 in, 1 out]
        n249 = for {
          tunnel: w2998 -> [w3011] mode=indexing
          tunnel: [w3009] -> w2991 mode=indexing
          tunnel: [w3009] -> w2996
          tunnel: w2995 -> [w3008]
          n250 = Unbundle By Name(w3011) -> ("DATE"=w3010:timestamp)
          n251 = Format Date/Time String(time format string (%c)=w3008, seconds (now)=w3010) -> (date/time string=w3009:string)  [unwired: 1 in]
        }
        n252 = Get Date/Time In Seconds() -> (seconds since 1Jan1904=w2994:timestamp)
        n253 = Format Date/Time String(time format string (%c)=w2995, seconds (now)=w2994) -> (date/time string=w2993:string)  [unwired: 1 in]
        n254 = local write "TO"(w2993) -> ()
        n255 = local write "INITAIL DATE FROM"(w2996) -> ()
        n256 = Insert Into Array(array=w2991, new element=w2993) -> (w2988:string[])  [unwired: 1 in]
        n257 = Sort 1D Array(array=w2988) -> (sorted array=w2987:string[])
        n258 = Insert Into Array(array=w2991, index=0, new element="BEGIN OF YEAR") -> (w2990:string[])
        n259 = property on="TO" class="CmbBox"("Strings[]"=w2987) -> ()  [unwired: 2 in, 2 out]
        n260 = property on="INITAIL DATE FROM" class="CmbBox"("Strings[]"=w2990) -> ()  [unwired: 2 in, 2 out]
      }
      event Timeout {
        n261 = event-data() -> ()  [unwired: 1 in, 3 out]
      }
    }
  }
